vi "Read Resource.vi"(8 "error in (no error)":errorcluster, 11 "Digital Delay Generator in":refnum<class "Digital Delay Generator.lvclass">) -> (0 "error out":errorcluster, 2 "Resource":string, 3 "Digital Delay Generator out":refnum<class "Digital Delay Generator.lvclass">)   [LabVIEW 2018, in "Digital Delay Generator.lvlib" / "Digital Delay Generator.lvclass"]
uses:
  Digital Delay Generator.lvclass
  Digital Delay Generator.lvclass/Digital Delay Generator.ctl
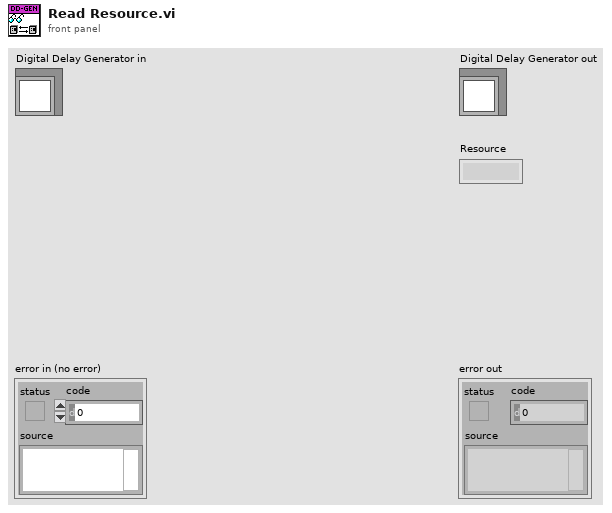
[diagram p1: front panel]
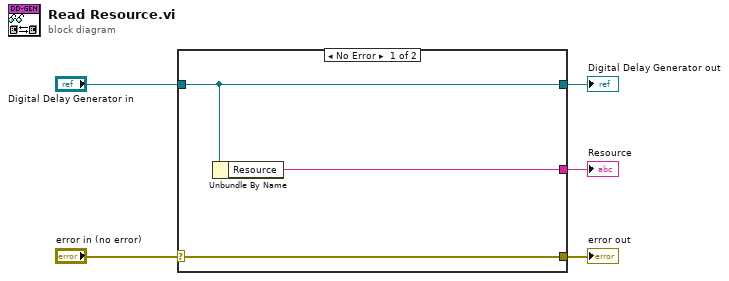
[diagram p0: block diagram]
diagram:
  n1 = case shown="No Error" "error in (no error)" {
    selector: "error in (no error)" -> [w8 w9]
    tunnel: [w8 w9] -> w4
    tunnel: [w7 w10] -> w2
    tunnel: "Digital Delay Generator in" -> [w7 w10]
    tunnel: [w6 _] -> w1
    frame No Error {
      n2 = Unbundle By Name(w7) -> ("Resource"=w6:string)
    }
    frame Error {
    }
  }
  "error out" <- w4
  "Digital Delay Generator out" <- w2
  "Resource" <- w1
